vi "{All}.vi"() -> (1 "Word":string)   [LabVIEW 2018, in "Application.lvlib" / "Keywords.lvclass"]
uses:
  Keywords.lvclass
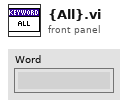
[diagram p1: front panel]
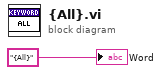
[diagram p0: block diagram]
diagram:
  "Word" <- "{All}"
